vi "Focus Image Stack.vi"(8 "error in (no error)":errorcluster, 10 "Kernel Size":i32, 11 "Image Stack":T1[](array[typedef])) -> (0 "error out":errorcluster, 2 "Height Map":T1(plugin-control), 3 "Focused Image":T1(plugin-control))   [LabVIEW 2013]
uses:
  <vilib>/vision/Image Controls.llb/IMAQ Image.ctl
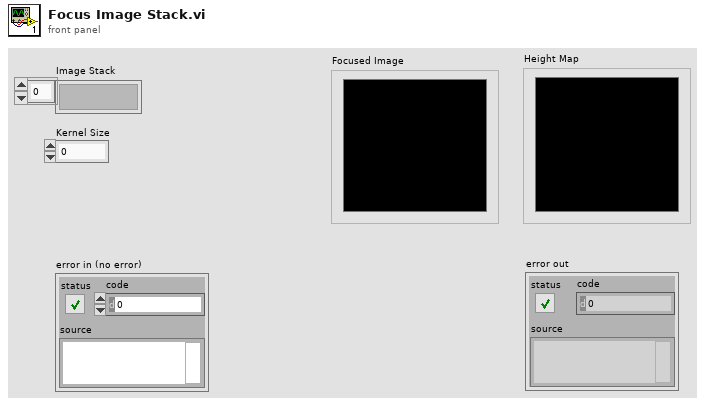
[diagram p1: front panel]
types:
  T1 = typedef "IMAQ Image.ctl" = refnum<image>
  T2 = typedef "Image Type" = u32
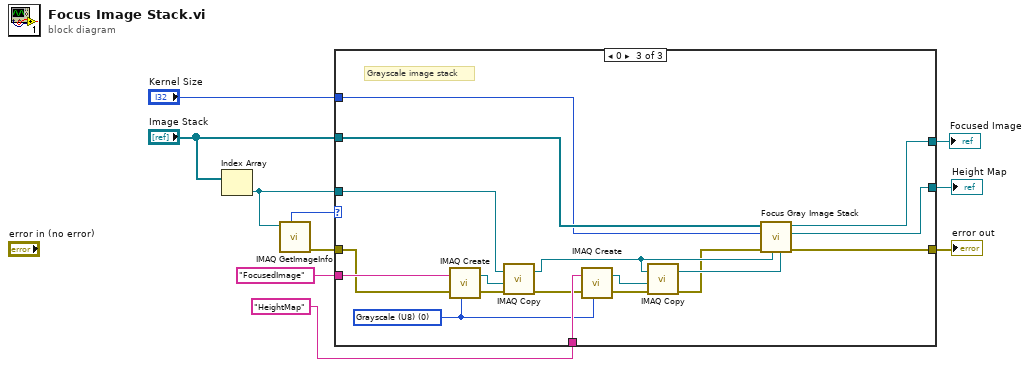
[diagram p0: block diagram]
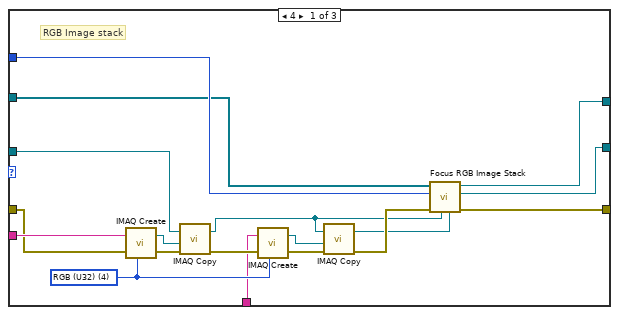
[diagram p2: hidden frame]
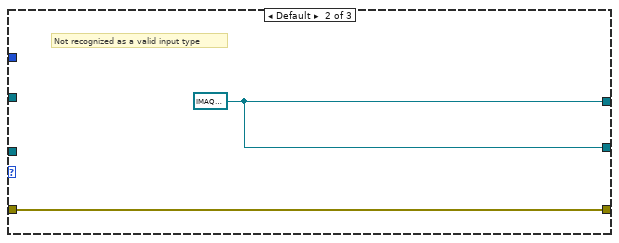
[diagram p3: hidden frame]
diagram:
  n1 = Index Array(array="Image Stack") -> (element=w1:T1)  [unwired: 1 in]
  n2 = call "IMAQ GetImageInfo"("Image"=w1) -> ("error out"=w10:errorcluster, "Image Type"=w9:T2)  [unwired: 3 in, 6 out]
  n3 = case shown="0" w9 {
    tunnel: w10 -> [w15 w30 w42]
    tunnel: [w26 w30 w48] -> w8
    tunnel: [w24 w29 w44] -> w7
    tunnel: [w25 w29 w45] -> w6
    tunnel: "Image Stack" -> [w27 _ w47]
    tunnel: "Kernel Size" -> [w28 _ w46]
    tunnel: "HeightMap" ("Image Name") -> [w16 _ w41]
    tunnel: "FocusedImage" ("Image Name") -> [w17 _ w43]
    tunnel: w1 -> [w13 _ w38]
    frame 4 {
      w23 = T2 4 items=["Grayscale (U8)", "Grayscale (I16)", "Grayscale (SGL)", "Complex (CSG)", "RGB (U32)", "HSL (U32)", "RGB (U64)", "Grayscale (U16)"] ("Image Type")
      # "RGB Image stack"
      n4 = call "IMAQ Create"("Image Name"=w17, "Image Type"=w23, "error in (no error)"=w15) -> ("New Image"=w21:T1, "error out"=w22:errorcluster)  [unwired: 2 in]
      n5 = call "IMAQ Copy"("error in (no error)"=w22, "Image Dst"=w21, "Image Src"=w13) -> ("error out"=w20:errorcluster, "Image Dst Out"=w12:T1)  [unwired: 3 in]
      n6 = call "IMAQ Create"("Image Name"=w16, "Image Type"=w23, "error in (no error)"=w20) -> ("New Image"=w18:T1, "error out"=w19:errorcluster)  [unwired: 2 in]
      n7 = call "IMAQ Copy"("error in (no error)"=w19, "Image Dst"=w18, "Image Src"=w12) -> ("error out"=w14:errorcluster, "Image Dst Out"=w11:T1)  [unwired: 3 in]
      n8 = call "Focus RGB Image Stack.vi"("Height Map"=w11, "Focused Image"=w12, "error in (no error)"=w14, "Kernel Size"=w28, "Image Stack"=w27) -> ("error out"=w26:errorcluster, "Height Map"=w24:T1, "Focused Image"=w25:T1)  [unwired: 4 in]
    }
    frame Default {
      w29 = T1 refnum ("Focused Image")
      # "Not recognized as a valid input type"
    }
    frame 0 {
      w40 = T2 0 items=["Grayscale (U8)", "Grayscale (I16)", "Grayscale (SGL)", "Complex (CSG)", "RGB (U32)", "HSL (U32)", "RGB (U64)", "Grayscale (U16)"] ("Image Type")
      # "Grayscale image stack"
      n9 = call "IMAQ Create"("Image Name"=w43, "Image Type"=w40, "error in (no error)"=w42) -> ("New Image"=w37:T1, "error out"=w39:errorcluster)  [unwired: 2 in]
      n10 = call "IMAQ Copy"("error in (no error)"=w39, "Image Dst"=w37, "Image Src"=w38) -> ("error out"=w36:errorcluster, "Image Dst Out"=w33:T1)  [unwired: 3 in]
      n11 = call "IMAQ Create"("Image Name"=w41, "Image Type"=w40, "error in (no error)"=w36) -> ("New Image"=w34:T1, "error out"=w35:errorcluster)  [unwired: 2 in]
      n12 = call "IMAQ Copy"("error in (no error)"=w35, "Image Dst"=w34, "Image Src"=w33) -> ("error out"=w31:errorcluster, "Image Dst Out"=w32:T1)  [unwired: 3 in]
      n13 = call "Focus Gray Image Stack.vi"("Height Map"=w32, "Focused Image"=w33, "error in (no error)"=w31, "Kernel Size"=w46, "Image Stack"=w47) -> ("error out"=w48:errorcluster, "Height Map"=w44:T1, "Focused Image"=w45:T1)  [unwired: 4 in]
    }
  }
  "error out" <- w8
  "Focused Image" <- w6
  "Height Map" <- w7
